vi "velocity_control.vi"(8 "pres_y":dbl, 9 "pres_x":dbl, 10 "pres_angle":dbl, 11 "totalForce":cdb[](array[numeric])) -> (1 "rad_right":dbl, 2 "rad_left":dbl)   [LabVIEW 2015]
uses:
  <vilib>/imath/engines/lvmath2/RunTimeEngine/IndexRead/NIMS V(S).vi
  <instcachedir>/0/NIMS V(S)_0488751826AF41519A22953C041130DC.lvgen/NIMS V(S)_0488751826AF41519A22953C041130DC_003.vi
  <vilib>/imath/engines/lvmath2/RunTimeEngine/BuiltInFunctions/atan2/NIMS_atan2.vi
  <instcachedir>/0/NIMS_atan2_A91AA4A7D42247EDBE8F76DB99AF04A4.lvgen/NIMS_atan2_A91AA4A7D42247EDBE8F76DB99AF04A4_001.vi
  <vilib>/imath/engines/lvmath2/RunTimeEngine/ErrorHandling/NIMS_Create Error From Enums.vi
  <vilib>/imath/engines/lvmath2/RunTimeEngine/CommandStatement/MC_CommandStatement_break.vi
  <vilib>/imath/engines/lvmath2/RunTimeEngine/CommandStatement/NIMS_CommandStatement_MaskErr.vi
  <vilib>/imath/engines/lvmath2/RunTimeEngine/VariableToken/NIMS_VariableToken_CondDefined.vi
  <instcachedir>/0/NIMS_VariableToken_CondDefined_FE30D0A1BFB24F098D41DEBABFE96BE1.lvgen/NIMS_VariableToken_CondDefined_FE30D0A1BFB24F098D41DEBABFE96BE1_005.vi
  <vilib>/imathl/engines/lvmath/Functions/Error Handling/Create Error.vi
  <vilib>/imath/engines/lvmath2/RunTimeEngine/NodeEndStatement/NIMS_NodeEndStatement_Output.vi
  <instcachedir>/0/NIMS_NodeEndStatement_Output_53EC0D466D134D7ABD903AC30B43404B.lvgen/NIMS_NodeEndStatement_Output_53EC0D466D134D7ABD903AC30B43404B_001.vi
  <vilib>/imath/engines/lvmath2/RunTimeEngine/ErrorHandling/NIMS_Finalize Error.vi
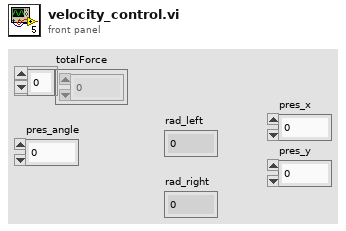
[diagram p1: front panel]
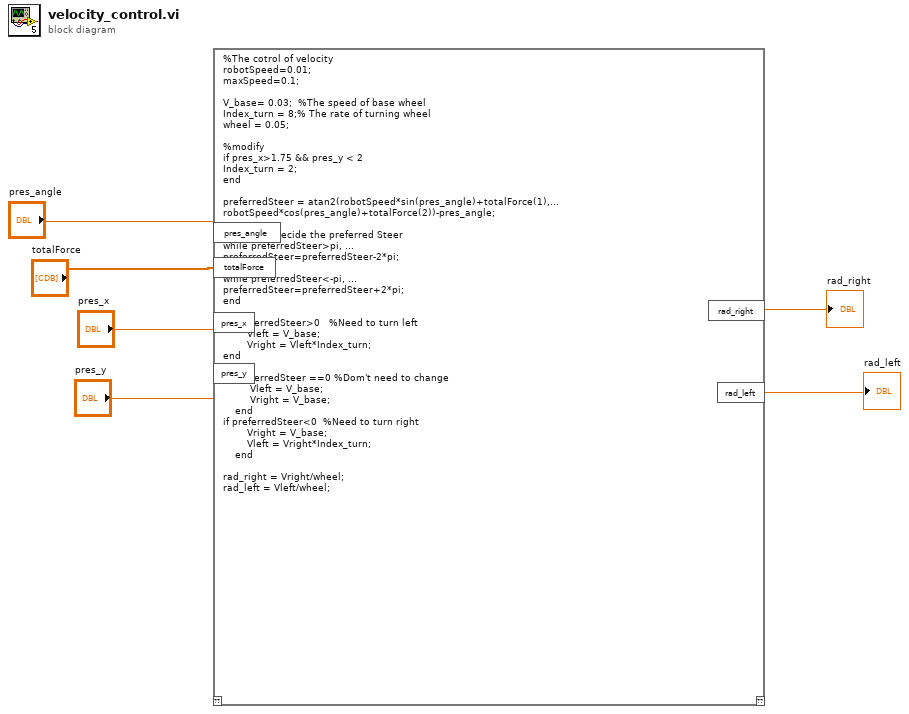
[diagram p0: block diagram]
diagram:
  n1 = mathscript code="%The cotrol of velocity\nrobotSpeed=0.01; \nmaxSpeed=0.1; \n\nV_base= 0.03;  %The speed of base wheel\nIndex_turn = 8;% The rate of turning wheel\nwheel = 0.05;\n\n%modify\nif pres_x>1.75 && pres_y < 2\nIndex_turn = 2;\nend\n\npreferredSteer = atan2(robotSpeed*sin(pres_angle)+totalForce(1),...\nrobotSpeed*cos(pres_angle)+totalForce(2))-pres_angle; \n \n%Judge to decide the preferred Steer\nwhile preferredSteer>pi, ...\npreferredSteer=preferredSteer-2*pi; \nend \nwhile preferredSteer<-pi, ...\npreferredSteer=preferredSteer+2*pi; \nend\n\n if preferredSteer>0   %Need to turn left\n        Vleft = V_base;\n        Vright = Vleft*Index_turn;\nend\n\n if preferredSteer ==0 %Dom't need to change\n         Vleft = V_base;\n         Vright = V_base;\n    end\nif preferredSteer<0  %Need to turn right\n        Vright = V_base;\n        Vleft = Vright*Index_turn;\n    end\n    \nrad_right = Vright/wheel;\nrad_left = Vleft/wheel;"("pres_angle"="pres_angle", "totalForce"="totalForce", "pres_x"="pres_x", "pres_y"="pres_y") -> ("rad_right"=→"rad_right":dbl, "rad_left"=→"rad_left":dbl)  [unwired: 1 in, 1 out]
